vi "WPI_CameraBackground Loop.vi"(11 "CameraDevRef":T1) -> ()   [LabVIEW 2017]
doc: "This VI acquires the image buffer from the camera MJPG stream at the configured fps rate. It notifies any waiting VIs and allows them to pick up the latest image. This allows the camera and robot vision loop to run at different rates. The 1011, camera is far more efficient using MJPGs, and generally, this is probably the better choice for the camera loop.\n \nThis software is licensed. Open the labview\\readme\\WPI Robotics Library Open Source License.txt file for more information."
uses:
  <vilib>/Rock Robotics/WPI/Camera/WPI_CameraDevRef.ctl
  <vilib>/Rock Robotics/WPI/Camera/WPI_CameraSettings Operations.ctl
  <vilib>/Rock Robotics/WPI/Camera/WPI_CameraSettings Read MJPG.ctl
  <vilib>/Rock Robotics/WPI/Camera/WPI_CameraImageSize.ctl
panel:
  out "connection ID":refnum<k5>
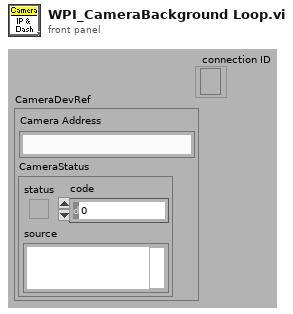
[diagram p1: front panel]
types:
  T1 = typedef "WPI_CameraDevRef.ctl" = cluster{"Camera Address":string, "CameraStatus":errorcluster}
  T2 = typedef "WPI_CameraSettings Operations.ctl" = enum16{"Udate FPS", "Update Compression", "Update Size", "Update White Balance", "Update Brightness", "Update Sharpness", "Update Exposure", "Update Exposure Value", "Update Color Level", "Update Exp Priority", "Update Color Enable", "Update JPG", "Update MJPG", "Read and Clear", "Read", "Init"}
  T3 = typedef "WPI_CameraSettings Read MJPG.ctl" = cluster{"fps":i32, "compression":i32, "Image Size":T4, "Config Shown":bool}
  T4 = typedef "WPI_CameraImageSize.ctl" = enum16{"640x480", "320x240", "160x120", "Custom"}
  T5 = typedef "WPI_CameraSettings Control.ctl" = cluster{"FPS":i32, "Compression":i32, "Size":i32, "White Balance":i32, "Brightness":i32, "Sharpness":i32, "Exposure":i32, "Color Level":i32, "Exposure Priority":i32, "Color Enable":i32, "JPG Loop":i32, "MJPG Loop":i32, "Exposure Value":i32}
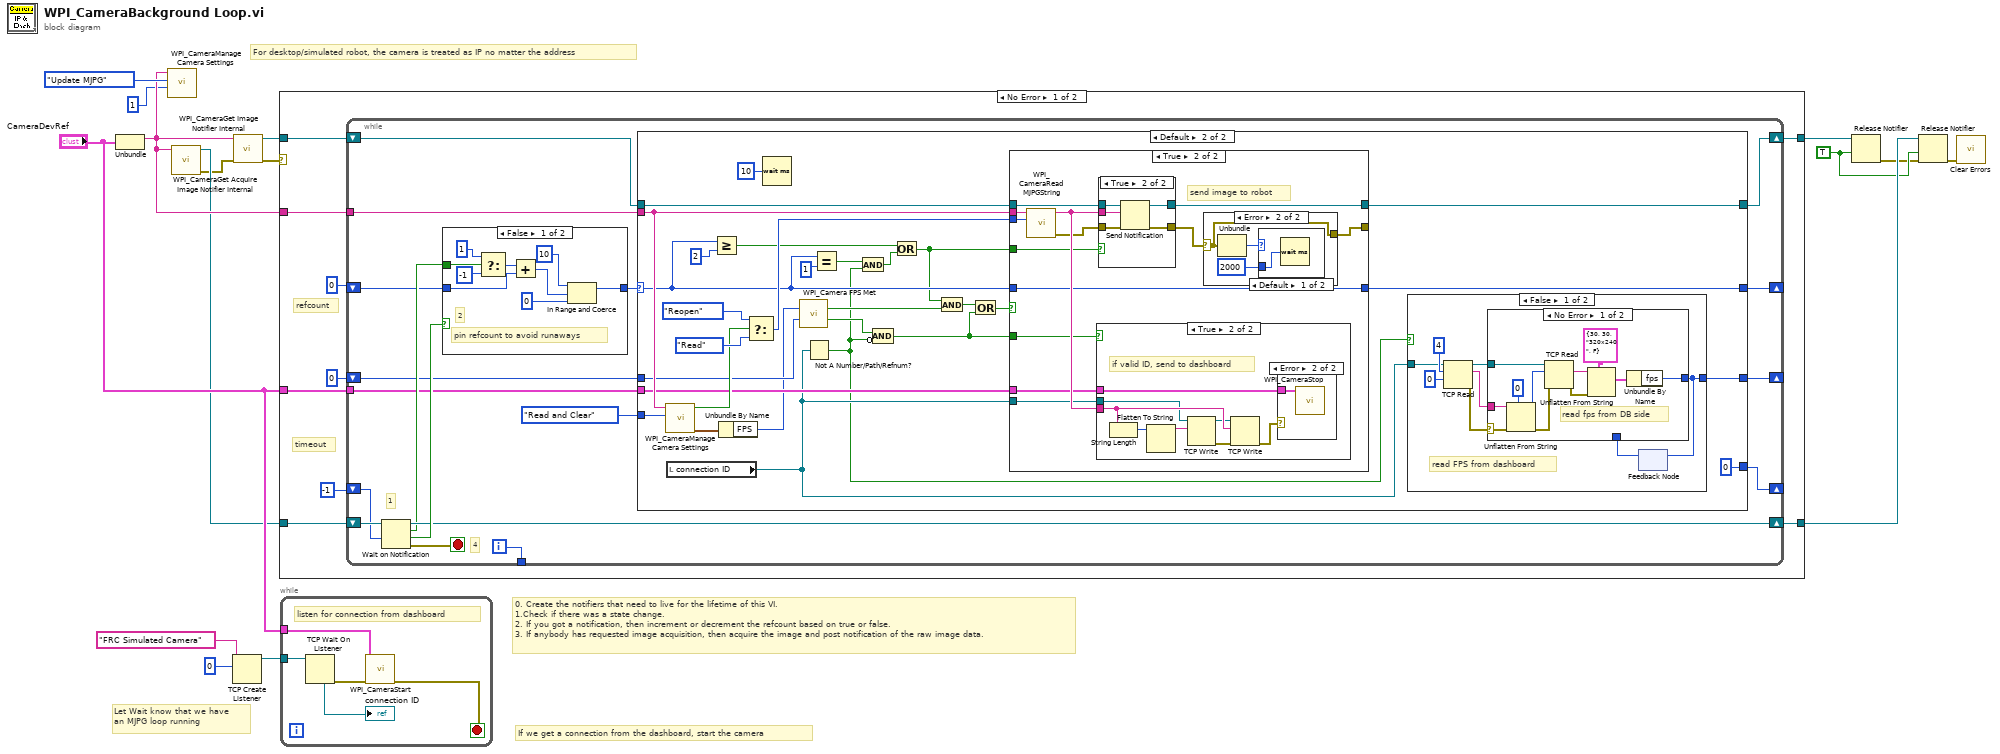
[diagram p0: block diagram]
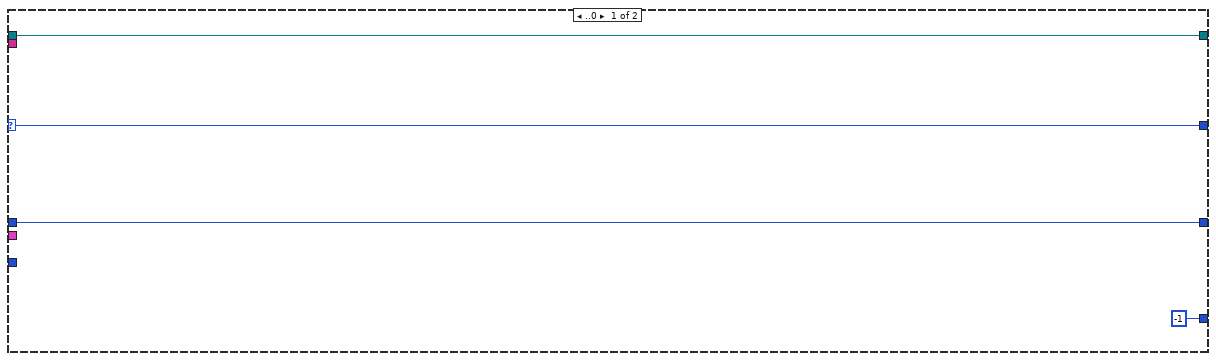
[diagram p2: hidden frame]
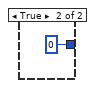
[diagram p4: hidden frame]
diagram:
  w10 = TRUE ("force destroy? (F)")
  # "For desktop/simulated robot, the camera is treated as IP no matter the address"
  # "If we get a connection from the dashboard, start the camera"
  # "Let Wait know that we have\nan MJPG loop running"
  # "0. Create the notifiers that need to live for the lifetime of this VI. \n1.Check if there was a state change.\n2. If you got a notification, then increment or decrement the refcount based on true or false.\n3. If anybody has requested image acquisition, then acquire the image and post notification of the raw image data."
  n1 = Unbundle("CameraDevRef") -> ("Camera Address"=w14:string)  [unwired: 1 out]
  n2 = call <vilib>:"WPI_CameraManage Camera Settings.vi"("Value"=1, "Operation"=WPI_CameraSettings_Operations."Update MJPG", "Camera IP"=w14) -> ()  [unwired: 7 in, 2 out]
  n3 = call <vilib>:"WPI_CameraGet Acquire Image Notifier Internal.vi"("Camera Address"=w14) -> ("error out"=w6:errorcluster, "Acquire Image Notifier"=w7:refnum<notifier>)  [unwired: 1 in, 8 out]
  n4 = TCP Create Listener(10:u16 0 ("port"), 11:"FRC Simulated Camera" ("service name")) -> (3:w3:refnum<k5>)  [unwired: 3 in, 2 out]
  n5 = call <vilib>:"WPI_CameraGet Image Notifier Internal.vi"("error in (no error)"=w6, "Camera Address"=w14) -> ("error out"=w9:errorcluster, "Image Notifier"=w11:refnum<notifier>)  [unwired: 8 out]
  n6 = case shown="No Error" w9 {
    tunnel: w14 -> [w25 _]
    tunnel: w7 -> [w24 w145]
    tunnel: w11 -> [w22 w146]
    tunnel: [w20 w146] -> w13
    tunnel: [w19 w145] -> w12
    tunnel: "CameraDevRef" -> [w18 _]
    frame No Error {
      # "timeout"
      # "refcount"
      n7 = while {
        shift-right: [w41] -> w19
        shift-left: w24 -> [w43]
        tunnel: w25 -> [w38]
        shift-right: [w31] -> _
        shift-left: 0 -> [w39]
        shift-right: [w36] -> w20
        shift-left: w22 -> [w37]
        shift-right: [w34] -> _
        shift-left: -1 -> [w35]
        tunnel: [w29] -> _
        tunnel: w18 -> [w28]
        shift-right: [w27] -> _
        shift-left: 0 ("fps") -> [w26]
        i -> [w29]
        stop <- w33 stop-if-true
        # "4"
        # "1"
        n8 = Wait on Notification(notifier=w43, timeout in ms (-1)=w35) -> (notifier out=w41:refnum<notifier>, notification=w40:bool, timed out?=w42:bool, error out=w33:errorcluster)  [unwired: 1 in, 1 out]
        n9 = case shown="False" w42 {
          tunnel: w40 -> [w143 _]
          tunnel: w39 -> [w139 w144]
          tunnel: [w135 w144] -> w32
          frame False {
            # "pin refcount to avoid runaways"
            # "2"
            n10 = Select(t=1, s=w143, f=-1) -> (s? t:f=w140:i32)
            n11 = Add(x=w140, y=w139) -> (x+y=w136:i32)
            n12 = In Range and Coerce(upper limit=10, x=w136, lower limit=0) -> (coerced(x)=w135:i32)  [unwired: 1 out]
          }
          frame True {
          }
        }
        n13 = case shown="Default" w32 {
          selector: w32 -> [w46 w53]
          tunnel: w38 -> [_ w68]
          tunnel: w37 -> [w47 w77]
          tunnel: [w47 w76] -> w36
          tunnel: [-1 0] -> w34
          tunnel: [w46 w62] -> w31
          tunnel: WPI_CameraSettings_Operations."Read and Clear" ("Operation") -> [_ w69]
          tunnel: w28 -> [_ w67]
          tunnel: [w44 w61] -> w27
          tunnel: w26 -> [w44 w65]
          frame ..0 {
          }
          frame Default {
            n14 = call <vilib>:"WPI_CameraManage Camera Settings.vi"("Operation"=w69, "Camera IP"=w68) -> ("Values"=w70:T5, "Changed"=w71:bool)  [unwired: 8 in]
            n15 = local read "connection ID"() -> (w60:refnum<k5>)
            n16 = Greater Or Equal?(x=w53, y=2) -> (x >= y?=w50:bool)
            n17 = Unbundle By Name(w70) -> ("FPS"=w64:i32)
            n18 = Select(t=enum16{"Read", "Reopen", "Close"}."Reopen" ("Operation"), s=w71, f=enum16{"Read", "Reopen", "Close"}."Read" ("Operation")) -> (s? t:f=w72:enum16{"Read", "Reopen", "Close"})
            n19 = Wait (ms)(milliseconds to wait=u32 10) -> ()  [unwired: 1 out]
            n20 = call <vilib>:"WPI_Camera FPS Met.vi"("robot fps"=w64, "dashboard fps"=w65) -> ("robot fps met?"=w54:bool, "dashboard fps met?"=w58:bool)  [unwired: 12 in]
            n21 = Not A Number/Path/Refnum?(number/path/refnum=w60) -> (NaN/Path/Refnum?=w48:bool)
            n22 = Equal?(x=w53, y=1) -> (x = y?=w56:bool)
            n23 = And(x=w56, y=w48) -> (x .and. y?=w51:bool)
            n24 = Compound Arithmetic op=AND(w58, invert w48) -> (w59:bool)
            n25 = Or(x=w50, y=w51) -> (x .or. y?=w49:bool)
            n26 = And(x=w49, y=w54) -> (x .and. y?=w55:bool)
            n27 = Or(x=w55, y=w59) -> (x .or. y?=w63:bool)
            n28 = case shown="True" w63 {
              tunnel: w77 -> [w100 w113]
              tunnel: [w100 w112] -> w76
              tunnel: [_ w101] -> _
              tunnel: w72 -> [_ w111]
              tunnel: w68 -> [_ w110]
              tunnel: w53 -> [w99 w106]
              tunnel: w60 -> [_ w108]
              tunnel: w67 -> [_ w107]
              tunnel: [w99 w106] -> w62
              tunnel: w59 -> [_ w105]
              tunnel: w49 -> [_ w104]
              frame False {
              }
              frame True {
                # "send image to robot"
                n29 = call <vilib>:"WPI_CameraRead MJPGString.vi"("Operation"=w111, "address"=w110) -> ("error out"=w103:errorcluster, "Raw Image Data"=w109:string)  [unwired: 8 in]
                n30 = case shown="True" w105 {
                  tunnel: w109 -> [_ w121]
                  tunnel: w108 -> [_ w118]
                  tunnel: w107 -> [_ w114]
                  frame False {
                  }
                  frame True {
                    # "if valid ID, send to dashboard"
                    n31 = String Length(string=w121) -> (length=w120:i32)
                    n32 = Flatten To String(anything=w120) -> (data string=w119:string)  [unwired: 3 in, 2 out]
                    n33 = TCP Write(connection ID=w118, data in=w119) -> (connection ID out=w115:refnum<k5>, error out=w117:errorcluster)  [unwired: 2 in, 1 out]
                    n34 = TCP Write(connection ID=w115, data in=w121, error in (no error)=w117) -> (error out=w116:errorcluster)  [unwired: 1 in, 2 out]
                    n35 = case shown="Error" w116 {
                      tunnel: w114 -> [_ w122]
                      frame No Error {
                      }
                      frame Error {
                        n36 = call <vilib>:"WPI_CameraStop.vi"("CameraDevRef"=w122) -> ()  [unwired: 1 in, 10 out]
                      }
                    }
                  }
                }
                n37 = case shown="True" w104 {
                  tunnel: w113 -> [w124 w129]
                  tunnel: [w124 w128] -> w112
                  tunnel: [w123 w127] -> w102
                  tunnel: w103 -> [w123 w126]
                  tunnel: w109 -> [_ w125]
                  frame False {
                  }
                  frame True {
                    n38 = Send Notification(notification=w125, notifier=w129, error in (no error)=w126) -> (notifier out=w128:refnum<notifier>, error out=w127:errorcluster)
                  }
                }
                n39 = case shown="Error" w102 {
                  selector: w102 -> [w130 w131]
                  tunnel: [w130 w131] -> w101
                  frame No Error {
                  }
                  frame Error {
                    n40 = Unbundle(w131) -> ("code"=w133:i32)  [unwired: 2 out]
                    n41 = case shown="Default" w133 {
                      tunnel: u32 2000 ("milliseconds to wait") -> [w134 _]
                      frame Default {
                        n42 = Wait (ms)(milliseconds to wait=w134) -> ()  [unwired: 1 out]
                      }
                      frame 56 {
                      }
                    }
                  }
                }
              }
            }
            n43 = case shown="False" w48 {
              tunnel: [w80 0 ("fps")] -> w61
              tunnel: w60 -> [w78 _]
              frame False {
                # "read FPS from dashboard"
                n44 = TCP Read(connection ID=w78, bytes to read=4, 9:0 ("timeout ms (25000)")) -> (connection ID out=w82:refnum<k5>, data out=w83:string, error out=w81:errorcluster)  [unwired: 2 in]
                n45 = feedback #1() -> (w79:i32)  [unwired: 1 in]
                n46 = case shown="No Error" w81 {
                  selector: w81 -> [w87 _]
                  tunnel: w83 -> [w95 _]
                  tunnel: w82 -> [w93 _]
                  tunnel: [w86 w97] -> w80
                  tunnel: w79 -> [_ w97]
                  frame No Error {
                    # "read fps from DB side"
                    n47 = Unflatten From String(type=0 ("bytes to read"), binary string=w95, error in (no error)=w87) -> (value=w92:i32, error out=w94:errorcluster)  [unwired: 2 in, 1 out]
                    n48 = TCP Read(connection ID=w93, bytes to read=w92, error in (no error)=w94) -> (data out=w91:string, error out=w90:errorcluster)  [unwired: 1 in, 2 out]
                    n49 = Unflatten From String(type=T3 {"fps"=30, "compression"=30, "Image Size"=enum."320x240", "Config Shown"=FALSE} ("Camera Settings"), binary string=w91, error in (no error)=w90) -> (value=w88:T3)  [unwired: 2 in, 2 out]
                    n50 = Unbundle By Name(w88) -> ("fps"=w86:i32)
                  }
                  frame Error {
                  }
                }
                n51 = feedback-in #1(w80) -> ()
              }
              frame True {
              }
            }
          }
        }
      }
    }
    frame Error {
    }
  }
  n52 = while {
    tunnel: w3 -> [w151]
    tunnel: "CameraDevRef" -> [w147]
    stop <- w148 stop-if-true
    # "listen for connection from dashboard"
    n53 = TCP Wait On Listener(11:w151) -> (0:w149:errorcluster, 4:→"connection ID":refnum<k5>)  [unwired: 3 in, 3 out]
    n54 = call <vilib>:"WPI_CameraStart.vi"("error in (no error)"=w149, "CameraDevRef"=w147) -> ("error out"=w148:errorcluster)  [unwired: 9 out]
  }
  n55 = Release Notifier(notifier=w13, force destroy? (F)=w10) -> (error out=w5:errorcluster)  [unwired: 1 in, 2 out]
  n56 = Release Notifier(notifier=w12, force destroy? (F)=w10, error in (no error)=w5) -> (error out=w8:errorcluster)  [unwired: 2 out]
  n57 = call <vilib>:"Clear Errors.vi"("error in (no error)"=w8) -> ()  [unwired: 1 in, 6 out]
